vi "Generate OD data.vi"(4 "dark":u16[][](array[numeric]), 5 "light":u16[][](array[numeric]), 6 "atom":u16[][](array[numeric])) -> (2 "OD image":dbl[][](array[numeric]))   [LabVIEW 2013]
panel:
  out "x*y":dbl[][](array[numeric])
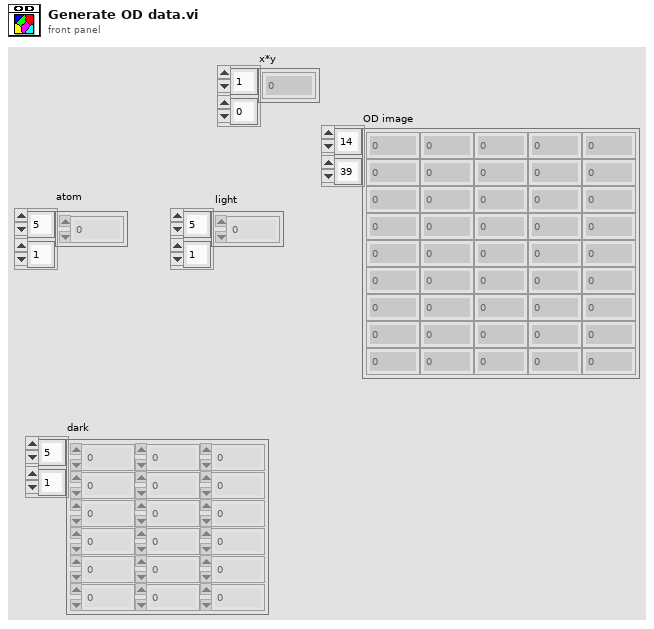
[diagram p1: front panel]
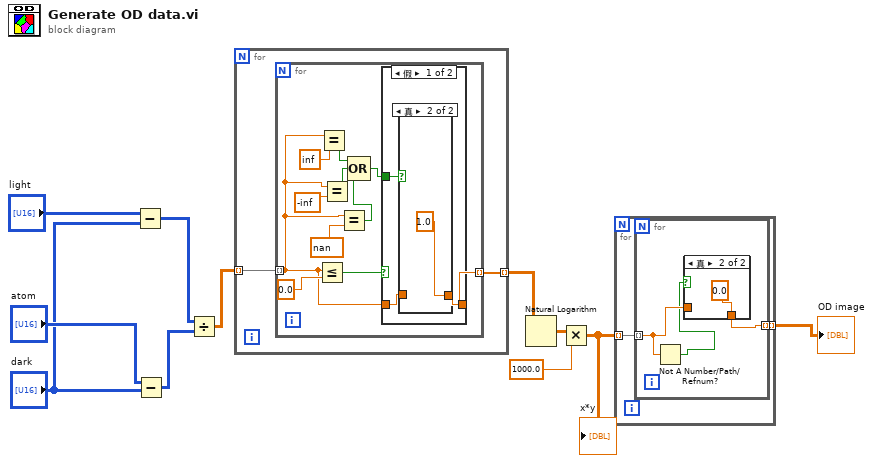
[diagram p0: block diagram]
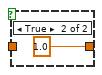
[diagram p4: hidden frame]
diagram:
  n1 = Subtract(x="light", y="dark") -> (x-y=w8:u16[][])
  n2 = Subtract(x="atom", y="dark") -> (x-y=w7:u16[][])
  n3 = Divide(x=w8, y=w7) -> (x/y=w6:dbl[][])
  n4 = for {
    tunnel: w6 -> [w13] mode=indexing
    tunnel: [w12] -> w5 mode=indexing
    n5 = for {
      tunnel: w13 -> [w18] mode=indexing
      tunnel: [w22] -> w12 mode=indexing
      n6 = Less Or Equal?(x=w18, y=0.0) -> (x <= y?=w23:bool)
      n7 = Equal?(x=w18, y=inf) -> (x = y?=w17:bool)
      n8 = Equal?(x=w18, y=-inf) -> (x = y?=w16:bool)
      n9 = Equal?(x=w18, y=nan) -> (x = y?=w15:bool)
      n10 = Compound Arithmetic op=OR(w17, w16, w15) -> (w14:bool)
      n11 = case shown="假" w23 {
        tunnel: w18 -> [w25 _]
        tunnel: [w26 1.0 ("数值")] -> w22
        tunnel: w14 -> [w27 _]
        frame False {
          n12 = case shown="真" w27 {
            tunnel: [w28 1.0 ("y")] -> w26
            tunnel: w25 -> [w28 _]
            frame False {
            }
            frame True {
            }
          }
        }
        frame True {
        }
      }
    }
  }
  n13 = Natural Logarithm(1:w5) -> (0:w3:dbl[][])
  n14 = Multiply(x=w3, y=1000.0) -> (x*y=w1:dbl[][])
  "x*y" <- w1
  n15 = for {
    tunnel: [w32] -> w2 mode=indexing
    tunnel: w1 -> [w31] mode=indexing
    n16 = for {
      tunnel: [w35] -> w32 mode=indexing
      tunnel: w31 -> [w34] mode=indexing
      n17 = Not A Number/Path/Refnum?(number/path/refnum=w34) -> (NaN/Path/Refnum?=w33:bool)
      n18 = case shown="真" w33 {
        tunnel: [w36 0.0 ("y")] -> w35
        tunnel: w34 -> [w36 _]
        frame False {
        }
        frame True {
        }
      }
    }
  }
  "OD image" <- w2
